vi "Write Return Q Setpoint Msg.vi"(10 "Return Q Setpoint Msg":refnum<class "Return Setpoint Msg.lvclass">, 11 "Optimization in":refnum<class "Optimization.lvclass">) -> (3 "Optimization out":refnum<class "Optimization.lvclass">)   [LabVIEW 2016, in "Optimization Framework.lvlib" / "Optimization.lvclass"]
uses:
  Optimization.lvclass
  Optimization Messages/Return Setpoint Msg/Return Setpoint Msg.lvclass
  Optimization.lvclass/Optimization.ctl
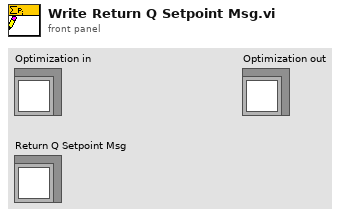
[diagram p1: front panel]
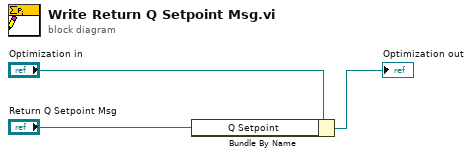
[diagram p0: block diagram]
diagram:
  n1 = Bundle By Name(cluster="Optimization in", "Q Setpoint"="Return Q Setpoint Msg") -> (→"Optimization out":refnum<class "Optimization.lvclass">)
